vi "Lab Panel V5.11.vi"() -> ()   [LabVIEW 2013] (continued)
                  frame #0 {
                    n2509 = Merge Signals(w4745, w4744) -> (→"LAB01 AMPS":dynamicdata)
                    n2510 = Merge Signals(w4742, w4741) -> (→"LAB01 VOLTS":dynamicdata)
                    n2511 = Merge Signals(w4722, w4721) -> (→"LAB03 VOLTS":dynamicdata)
                    n2512 = Merge Signals(w4739, w4738, w4737, w4736) -> (→"LAB01 deg C":dynamicdata)
                    n2513 = Merge Signals(w4735, w4734) -> (→"LAB02 AMPS":dynamicdata)
                    n2514 = Merge Signals(w4728, w4727, w4726, w4725) -> (→"LAB02 deg C":dynamicdata)
                    n2515 = Merge Signals(w4720, w4719, w4718, w4717) -> (→"LAB03 deg C":dynamicdata)
                    n2516 = Merge Signals(w4732, w4731) -> (→"LAB02 VOLTS":dynamicdata)
                    n2517 = Merge Signals(w4724, w4723) -> (→"LAB03 AMPS":dynamicdata)
                  }
                  frame #1 {
                    n2518 = Merge Signals(w4755, w4754) -> (→"LAB05 VOLTS":dynamicdata)
                    n2519 = Merge Signals(w4768, w4767) -> (→"LAB04 AMPS":dynamicdata)
                    n2520 = Merge Signals(w4757, w4756) -> (→"LAB05 AMPS":dynamicdata)
                    n2521 = Merge Signals(w4753, w4752, w4751, w4750) -> (→"LAB05 deg C":dynamicdata)
                    n2522 = Merge Signals(w4764, w4763, w4762, w4761) -> (→"LAB04 deg C":dynamicdata)
                    n2523 = Merge Signals(w4766, w4765) -> (→"LAB04 VOLTS":dynamicdata)
                  }
                  frame #2 {
                    n2524 = local read "LAB05 VOLTS"() -> (w4776:dynamicdata)
                    n2525 = local read "LAB04 VOLTS"() -> (w4777:dynamicdata)
                    n2526 = local read "LAB02 VOLTS"() -> (w4779:dynamicdata)
                    n2527 = local read "LAB03 VOLTS"() -> (w4778:dynamicdata)
                    n2528 = local read "LAB05 AMPS"() -> (w4782:dynamicdata)
                    n2529 = local read "LAB01 VOLTS"() -> (w4780:dynamicdata)
                    n2530 = local read "LAB04 AMPS"() -> (w4783:dynamicdata)
                    n2531 = local read "LAB03 AMPS"() -> (w4784:dynamicdata)
                    n2532 = local read "LAB03 deg C"() -> (w4772:dynamicdata)
                    n2533 = local read "LAB02 AMPS"() -> (w4785:dynamicdata)
                    n2534 = local read "LAB04 deg C"() -> (w4771:dynamicdata)
                    n2535 = local read "LAB05 deg C"() -> (w4770:dynamicdata)
                    n2536 = local read "LAB02 deg C"() -> (w4773:dynamicdata)
                    n2537 = local read "LAB01 deg C"() -> (w4774:dynamicdata)
                    n2538 = local read "LAB01 AMPS"() -> (w4786:dynamicdata)
                    n2539 = Merge Signals(w4774, w4773, w4772, w4771, w4770) -> (w4769:dynamicdata)
                    n2540 = Merge Signals(w4786, w4785, w4784, w4783, w4782) -> (w4781:dynamicdata)
                    n2541 = Merge Signals(w4780, w4779, w4778, w4777, w4776) -> (w4775:dynamicdata)
                    n2542 = global write "Global display 3.vi" "graph volts"(w4775) -> ()
                    n2543 = global write "Global display 3.vi" "graph deg C"(w4769) -> ()
                    n2544 = global write "Global display 3.vi" "graph amps"(w4781) -> ()
                  }
                }
              }
            }
          }
          frame #14 {
            # "check for amps fail"
            # "check for cycle test & temperature rise fail conditions"
            n2545 = local read "on loops"() -> (w4813:dbl)
            n2546 = local read "jig cycle"() -> (w4810:dbl)
            n2547 = local read "jig cycle"() -> (w4815:dbl)
            n2548 = Add(x=w4813, y=3.0) -> (x+y=w4811:dbl)
            n2549 = Equal?(x=w4810, y=w4811) -> (x = y?=w4806:bool)
            n2550 = local read "Fail Loops"() -> (w4787:dbl)
            n2551 = Equal?(x=w4815, y=1.0) -> (x = y?=w4808:bool)
            n2552 = global write "Global 1.vi" "fail count"(w4787) -> ()
            n2553 = stacked-sequence {
              tunnel: w4809 -> [w4818 _ _ _ _ _ _ _ _ _]
              tunnel: w4808 -> [w4819 w4839 w4859 w4879 w4899 w4919 w4939 w4959 w4979 w4999]
              tunnel: w4807 -> [w4816 _ _ _ _ _ _ _ _ _]
              tunnel: w4806 -> [w4817 w4838 w4858 w4878 w4898 w4918 w4938 w4958 w4978 w4998]
              tunnel: w4805 -> [_ w4837 _ _ _ _ _ _ _ _]
              tunnel: w4804 -> [_ w4836 _ _ _ _ _ _ _ _]
              tunnel: w4803 -> [_ _ w4857 _ _ _ _ _ _ _]
              tunnel: w4802 -> [_ _ w4856 _ _ _ _ _ _ _]
              tunnel: w4801 -> [_ _ _ w4877 _ _ _ _ _ _]
              tunnel: w4800 -> [_ _ _ w4876 _ _ _ _ _ _]
              tunnel: w4799 -> [_ _ _ _ w4897 _ _ _ _ _]
              tunnel: w4798 -> [_ _ _ _ w4896 _ _ _ _ _]
              tunnel: w4797 -> [_ _ _ _ _ w4917 _ _ _ _]
              tunnel: w4796 -> [_ _ _ _ _ w4916 _ _ _ _]
              tunnel: w4795 -> [_ _ _ _ _ _ w4937 _ _ _]
              tunnel: w4794 -> [_ _ _ _ _ _ w4936 _ _ _]
              tunnel: w4793 -> [_ _ _ _ _ _ _ w4957 _ _]
              tunnel: w4792 -> [_ _ _ _ _ _ _ w4956 _ _]
              tunnel: w4791 -> [_ _ _ _ _ _ _ _ w4977 _]
              tunnel: w4790 -> [_ _ _ _ _ _ _ _ w4976 _]
              tunnel: w4789 -> [_ _ _ _ _ _ _ _ _ w4997]
              tunnel: w4788 -> [_ _ _ _ _ _ _ _ _ w4996]
              frame #0 {
                # "LAB01-1"
                n2554 = case shown="True" w4816 {
                  tunnel: w4819 -> [_ w4832]
                  tunnel: w4818 -> [_ w4829]
                  tunnel: w4817 -> [_ w4828]
                  frame False {
                  }
                  frame True {
                    n2555 = local read "TEMP START LAB01-1"() -> (w4834:cluster{"TL":dbl, "TN":dbl})
                    n2556 = local read "RESULT LAB01-1"() -> (w4823:bool)
                    n2557 = local read "FAIL LAB01-1"() -> (w4826:cluster{"LO":dbl, "HI":dbl})
                    n2558 = local read "TDMS LAB01-1"() -> (w4833:refnum<k34>)
                    n2559 = local read "SET LAB01-1"() -> (w4830:T5)
                    n2560 = local read "DISP LAB01-1"() -> (w4831:T4)
                    n2561 = local read "SIG LAB01-1"() -> (w4835:T2)
                    n2562 = Bundle("FAIL LAB01-1"=w4826, "SIG LAB01-1"=w4835, "TEMP START LAB01-1"=w4834, "DISP LAB01-1"=w4831, "SET LAB01-1"=w4830, "TDMS LAB01-1"=w4833) -> (w4820:T32)  [unwired: 1 in]
                    n2563 = call "sub vi - cycle&temp fail v7.vi"("Amps Lo?"=w4832, "Input Cluster"=w4820, "SELECT"=w4829, "Amps Hi?"=w4828, "Result In"=w4823) -> ("(FAIL) out"=w4825:cluster{"FAIL LO":dbl, "FAIL HI":dbl}, "(DISP) out"=w4821:T4, "T-RISE"=w4822:cluster{"T-RISE (L)":dbl, "T-RISE (N)":dbl}, "Result Out"=w4824:bool, "file error"=w4827:errorcluster)  [unwired: 10 in]
                    n2564 = local write "TEMP RISE LAB01-1"(w4822) -> ()
                    n2565 = local write "FAIL LAB01-1"(w4825) -> ()
                    n2566 = local write "DISP LAB01-1"(w4821) -> ()
                    n2567 = local write "RESULT LAB01-1"(w4824) -> ()
                    n2568 = local write "data file error"(w4827) -> ()
                  }
                }
              }
              frame #1 {
                # "LAB01-2"
                n2569 = case shown="True" w4837 {
                  tunnel: w4839 -> [_ w4852]
                  tunnel: w4836 -> [_ w4849]
                  tunnel: w4838 -> [_ w4848]
                  frame False {
                  }
                  frame True {
                    n2570 = local read "TEMP START LAB01-2"() -> (w4854:cluster{"TL":dbl, "TN":dbl})
                    n2571 = local read "FAIL LAB01-2"() -> (w4845:cluster{"LO":dbl, "HI":dbl})
                    n2572 = local read "TDMS LAB01-2"() -> (w4853:refnum<k34>)
                    n2573 = local read "SET LAB01-2"() -> (w4850:T5)
                    n2574 = local read "DISP LAB01-2"() -> (w4851:T4)
                    n2575 = local read "RESULT LAB01-2"() -> (w4842:bool)
                    n2576 = local read "SIG LAB01-2"() -> (w4855:T2)
                    n2577 = Bundle("FAIL LAB01-2"=w4845, "SIG LAB01-2"=w4855, "TEMP START LAB01-2"=w4854, "DISP LAB01-2"=w4851, "SET LAB01-2"=w4850, "TDMS LAB01-2"=w4853) -> (w4840:T33)  [unwired: 1 in]
                    n2578 = call "sub vi - cycle&temp fail v7.vi"("Amps Lo?"=w4852, "Input Cluster"=w4840, "SELECT"=w4849, "Amps Hi?"=w4848, "Result In"=w4842) -> ("(FAIL) out"=w4844:cluster{"FAIL LO":dbl, "FAIL HI":dbl}, "(DISP) out"=w4847:T4, "T-RISE"=w4841:cluster{"T-RISE (L)":dbl, "T-RISE (N)":dbl}, "Result Out"=w4843:bool, "file error"=w4846:errorcluster)  [unwired: 10 in]
                    n2579 = local write "TEMP RISE LAB01-2"(w4841) -> ()
                    n2580 = local write "FAIL LAB01-2"(w4844) -> ()
                    n2581 = local write "DISP LAB01-2"(w4847) -> ()
                    n2582 = local write "RESULT LAB01-2"(w4843) -> ()
                    n2583 = local write "data file error"(w4846) -> ()
                  }
                }
              }
              frame #2 {
                # "LAB02-1"
                n2584 = case shown="True" w4857 {
                  tunnel: w4859 -> [_ w4872]
                  tunnel: w4856 -> [_ w4869]
                  tunnel: w4858 -> [_ w4868]
                  frame False {
                  }
                  frame True {
                    n2585 = local read "TEMP START LAB02-1"() -> (w4874:cluster{"TL":dbl, "TN":dbl})
                    n2586 = local read "FAIL LAB02-1"() -> (w4865:cluster{"LO":dbl, "HI":dbl})
                    n2587 = local read "TDMS LAB02-1"() -> (w4873:refnum<k34>)
                    n2588 = local read "SET LAB02-1"() -> (w4870:T5)
                    n2589 = local read "DISP LAB02-1"() -> (w4871:T4)
                    n2590 = local read "SIG LAB02-1"() -> (w4875:T2)
                    n2591 = local read "RESULT LAB02-1"() -> (w4862:bool)
                    n2592 = Bundle("FAIL LAB02-1"=w4865, "SIG LAB02-1"=w4875, "TEMP START LAB02-1"=w4874, "DISP LAB02-1"=w4871, "SET LAB02-1"=w4870, "TDMS LAB02-1"=w4873) -> (w4860:T34)  [unwired: 1 in]
                    n2593 = call "sub vi - cycle&temp fail v7.vi"("Amps Lo?"=w4872, "Input Cluster"=w4860, "SELECT"=w4869, "Amps Hi?"=w4868, "Result In"=w4862) -> ("(FAIL) out"=w4864:cluster{"FAIL LO":dbl, "FAIL HI":dbl}, "(DISP) out"=w4867:T4, "T-RISE"=w4861:cluster{"T-RISE (L)":dbl, "T-RISE (N)":dbl}, "Result Out"=w4863:bool, "file error"=w4866:errorcluster)  [unwired: 10 in]
                    n2594 = local write "TEMP RISE LAB02-1"(w4861) -> ()
                    n2595 = local write "FAIL LAB02-1"(w4864) -> ()
                    n2596 = local write "DISP LAB02-1"(w4867) -> ()
                    n2597 = local write "RESULT LAB02-1"(w4863) -> ()
                    n2598 = local write "data file error"(w4866) -> ()
                  }
                }
              }
              frame #3 {
                # "LAB02-2"
                n2599 = case shown="True" w4877 {
                  tunnel: w4879 -> [_ w4892]
                  tunnel: w4876 -> [_ w4889]
                  tunnel: w4878 -> [_ w4888]
                  frame False {
                  }
                  frame True {
                    n2600 = local read "TEMP START LAB02-2"() -> (w4894:cluster{"TL":dbl, "TN":dbl})
                    n2601 = local read "FAIL LAB02-2"() -> (w4885:cluster{"LO":dbl, "HI":dbl})
                    n2602 = local read "TDMS LAB02-2"() -> (w4893:refnum<k34>)
                    n2603 = local read "SET LAB02-2"() -> (w4890:T5)
                    n2604 = local read "DISP LAB02-2"() -> (w4891:T4)
                    n2605 = local read "SIG LAB02-2"() -> (w4895:T2)
                    n2606 = local read "RESULT LAB02-2"() -> (w4882:bool)
                    n2607 = Bundle("FAIL LAB02-2"=w4885, "SIG LAB02-2"=w4895, "TEMP START LAB02-2"=w4894, "DISP LAB02-2"=w4891, "SET LAB02-2"=w4890, "TDMS LAB02-2"=w4893) -> (w4880:T35)  [unwired: 1 in]
                    n2608 = call "sub vi - cycle&temp fail v7.vi"("Amps Lo?"=w4892, "Input Cluster"=w4880, "SELECT"=w4889, "Amps Hi?"=w4888, "Result In"=w4882) -> ("(FAIL) out"=w4884:cluster{"FAIL LO":dbl, "FAIL HI":dbl}, "(DISP) out"=w4887:T4, "T-RISE"=w4881:cluster{"T-RISE (L)":dbl, "T-RISE (N)":dbl}, "Result Out"=w4883:bool, "file error"=w4886:errorcluster)  [unwired: 10 in]
                    n2609 = local write "TEMP RISE LAB02-2"(w4881) -> ()
                    n2610 = local write "FAIL LAB02-2"(w4884) -> ()
                    n2611 = local write "DISP LAB02-2"(w4887) -> ()
                    n2612 = local write "RESULT LAB02-2"(w4883) -> ()
                    n2613 = local write "data file error"(w4886) -> ()
                  }
                }
              }
              frame #4 {
                # "LAB03-1"
                n2614 = case shown="True" w4897 {
                  tunnel: w4899 -> [_ w4912]
                  tunnel: w4896 -> [_ w4909]
                  tunnel: w4898 -> [_ w4908]
                  frame False {
                  }
                  frame True {
                    n2615 = local read "TEMP START LAB03-1"() -> (w4914:cluster{"TL":dbl, "TN":dbl})
                    n2616 = local read "FAIL LAB03-1"() -> (w4905:cluster{"LO":dbl, "HI":dbl})
                    n2617 = local read "TDMS LAB03-1"() -> (w4913:refnum<k34>)
                    n2618 = local read "SET LAB03-1"() -> (w4910:T5)
                    n2619 = local read "DISP LAB03-1"() -> (w4911:T4)
                    n2620 = local read "SIG LAB03-1"() -> (w4915:T2)
                    n2621 = local read "RESULT LAB03-1"() -> (w4902:bool)
                    n2622 = Bundle("FAIL LAB03-1"=w4905, "SIG LAB03-1"=w4915, "TEMP START LAB03-1"=w4914, "DISP LAB03-1"=w4911, "SET LAB03-1"=w4910, "TDMS LAB03-1"=w4913) -> (w4900:T36)  [unwired: 1 in]
                    n2623 = call "sub vi - cycle&temp fail v7.vi"("Amps Lo?"=w4912, "Input Cluster"=w4900, "SELECT"=w4909, "Amps Hi?"=w4908, "Result In"=w4902) -> ("(FAIL) out"=w4904:cluster{"FAIL LO":dbl, "FAIL HI":dbl}, "(DISP) out"=w4907:T4, "T-RISE"=w4901:cluster{"T-RISE (L)":dbl, "T-RISE (N)":dbl}, "Result Out"=w4903:bool, "file error"=w4906:errorcluster)  [unwired: 10 in]
                    n2624 = local write "TEMP RISE LAB03-1"(w4901) -> ()
                    n2625 = local write "FAIL LAB03-1"(w4904) -> ()
                    n2626 = local write "DISP LAB03-1"(w4907) -> ()
                    n2627 = local write "RESULT LAB03-1"(w4903) -> ()
                    n2628 = local write "data file error"(w4906) -> ()
                  }
                }
              }
              frame #5 {
                # "LAB03-2"
                n2629 = case shown="True" w4917 {
                  tunnel: w4919 -> [_ w4932]
                  tunnel: w4916 -> [_ w4929]
                  tunnel: w4918 -> [_ w4928]
                  frame False {
                  }
                  frame True {
                    n2630 = local read "TEMP START LAB03-2"() -> (w4934:cluster{"TL":dbl, "TN":dbl})
                    n2631 = local read "FAIL LAB03-2"() -> (w4925:cluster{"LO":dbl, "HI":dbl})
                    n2632 = local read "TDMS LAB03-2"() -> (w4933:refnum<k34>)
                    n2633 = local read "SET LAB03-2"() -> (w4930:T5)
                    n2634 = local read "DISP LAB03-2"() -> (w4931:T4)
                    n2635 = local read "RESULT LAB03-2"() -> (w4922:bool)
                    n2636 = local read "SIG LAB03-2"() -> (w4935:T2)
                    n2637 = Bundle("FAIL LAB03-2"=w4925, "SIG LAB03-2"=w4935, "TEMP START LAB03-2"=w4934, "DISP LAB03-2"=w4931, "SET LAB03-2"=w4930, "TDMS LAB03-2"=w4933) -> (w4920:T37)  [unwired: 1 in]
                    n2638 = call "sub vi - cycle&temp fail v7.vi"("Amps Lo?"=w4932, "Input Cluster"=w4920, "SELECT"=w4929, "Amps Hi?"=w4928, "Result In"=w4922) -> ("(FAIL) out"=w4924:cluster{"FAIL LO":dbl, "FAIL HI":dbl}, "(DISP) out"=w4927:T4, "T-RISE"=w4921:cluster{"T-RISE (L)":dbl, "T-RISE (N)":dbl}, "Result Out"=w4923:bool, "file error"=w4926:errorcluster)  [unwired: 10 in]
                    n2639 = local write "FAIL LAB03-2"(w4924) -> ()
                    n2640 = local write "TEMP RISE LAB03-2"(w4921) -> ()
                    n2641 = local write "DISP LAB03-2"(w4927) -> ()
                    n2642 = local write "RESULT LAB03-2"(w4923) -> ()
                    n2643 = local write "data file error"(w4926) -> ()
                  }
                }
              }
              frame #6 {
                # "LAB04-1"
                n2644 = case shown="True" w4937 {
                  tunnel: w4939 -> [_ w4952]
                  tunnel: w4936 -> [_ w4949]
                  tunnel: w4938 -> [_ w4948]
                  frame False {
                  }
                  frame True {
                    n2645 = local read "TEMP START LAB04-1"() -> (w4954:cluster{"TL":dbl, "TN":dbl})
                    n2646 = local read "FAIL LAB04-1"() -> (w4945:cluster{"LO":dbl, "HI":dbl})
                    n2647 = local read "TDMS LAB04-1"() -> (w4953:refnum<k34>)
                    n2648 = local read "SET LAB04-1"() -> (w4950:T5)
                    n2649 = local read "DISP LAB04-1"() -> (w4951:T4)
                    n2650 = local read "SIG LAB04-1"() -> (w4955:T2)
                    n2651 = local read "RESULT LAB04-1"() -> (w4942:bool)
                    n2652 = Bundle("FAIL LAB04-1"=w4945, "SIG LAB04-1"=w4955, "TEMP START LAB04-1"=w4954, "DISP LAB04-1"=w4951, "SET LAB04-1"=w4950, "TDMS LAB04-1"=w4953) -> (w4940:T38)  [unwired: 1 in]
                    n2653 = call "sub vi - cycle&temp fail v7.vi"("Amps Lo?"=w4952, "Input Cluster"=w4940, "SELECT"=w4949, "Amps Hi?"=w4948, "Result In"=w4942) -> ("(FAIL) out"=w4944:cluster{"FAIL LO":dbl, "FAIL HI":dbl}, "(DISP) out"=w4947:T4, "T-RISE"=w4941:cluster{"T-RISE (L)":dbl, "T-RISE (N)":dbl}, "Result Out"=w4943:bool, "file error"=w4946:errorcluster)  [unwired: 10 in]
                    n2654 = local write "TEMP RISE LAB04-1"(w4941) -> ()
                    n2655 = local write "FAIL LAB04-1"(w4944) -> ()
                    n2656 = local write "DISP LAB04-1"(w4947) -> ()
                    n2657 = local write "RESULT LAB04-1"(w4943) -> ()
                    n2658 = local write "data file error"(w4946) -> ()
                  }
                }
              }
              frame #7 {
                # "LAB04-2"
                n2659 = case shown="True" w4957 {
                  tunnel: w4959 -> [_ w4972]
                  tunnel: w4956 -> [_ w4969]
                  tunnel: w4958 -> [_ w4968]
                  frame False {
                  }
                  frame True {
                    n2660 = local read "TEMP START LAB04-2"() -> (w4974:cluster{"TL":dbl, "TN":dbl})
                    n2661 = local read "FAIL LAB04-2"() -> (w4965:cluster{"LO":dbl, "HI":dbl})
                    n2662 = local read "TDMS LAB04-2"() -> (w4973:refnum<k34>)
                    n2663 = local read "SET LAB04-2"() -> (w4970:T5)
                    n2664 = local read "DISP LAB04-2"() -> (w4971:T4)
                    n2665 = local read "SIG LAB04-2"() -> (w4975:T2)
                    n2666 = local read "RESULT LAB04-2"() -> (w4962:bool)
                    n2667 = Bundle("FAIL LAB04-2"=w4965, "SIG LAB04-2"=w4975, "TEMP START LAB04-2"=w4974, "DISP LAB04-2"=w4971, "SET LAB04-2"=w4970, "TDMS LAB04-2"=w4973) -> (w4960:T39)  [unwired: 1 in]
                    n2668 = call "sub vi - cycle&temp fail v7.vi"("Amps Lo?"=w4972, "Input Cluster"=w4960, "SELECT"=w4969, "Amps Hi?"=w4968, "Result In"=w4962) -> ("(FAIL) out"=w4964:cluster{"FAIL LO":dbl, "FAIL HI":dbl}, "(DISP) out"=w4967:T4, "T-RISE"=w4961:cluster{"T-RISE (L)":dbl, "T-RISE (N)":dbl}, "Result Out"=w4963:bool, "file error"=w4966:errorcluster)  [unwired: 10 in]
                    n2669 = local write "TEMP RISE LAB04-2"(w4961) -> ()
                    n2670 = local write "FAIL LAB04-2"(w4964) -> ()
                    n2671 = local write "DISP LAB04-2"(w4967) -> ()
                    n2672 = local write "RESULT LAB04-2"(w4963) -> ()
                    n2673 = local write "data file error"(w4966) -> ()
                  }
                }
              }
              frame #8 {
                # "LAB05-1"
                n2674 = case shown="True" w4977 {
                  tunnel: w4979 -> [_ w4992]
                  tunnel: w4976 -> [_ w4989]
                  tunnel: w4978 -> [_ w4988]
                  frame False {
                  }
                  frame True {
                    n2675 = local read "TEMP START LAB05-1"() -> (w4994:cluster{"TL":dbl, "TN":dbl})
                    n2676 = local read "FAIL LAB05-1"() -> (w4985:cluster{"LO":dbl, "HI":dbl})
                    n2677 = local read "TDMS LAB05-1"() -> (w4993:refnum<k34>)
                    n2678 = local read "SET LAB05-1"() -> (w4990:T5)
                    n2679 = local read "DISP LAB05-1"() -> (w4991:T4)
                    n2680 = local read "SIG LAB05-1"() -> (w4995:T2)
                    n2681 = local read "RESULT LAB05-1"() -> (w4982:bool)
                    n2682 = Bundle("FAIL LAB05-1"=w4985, "SIG LAB05-1"=w4995, "TEMP START LAB05-1"=w4994, "DISP LAB05-1"=w4991, "SET LAB05-1"=w4990, "TDMS LAB05-1"=w4993) -> (w4980:T40)  [unwired: 1 in]
                    n2683 = call "sub vi - cycle&temp fail v7.vi"("Amps Lo?"=w4992, "Input Cluster"=w4980, "SELECT"=w4989, "Amps Hi?"=w4988, "Result In"=w4982) -> ("(FAIL) out"=w4984:cluster{"FAIL LO":dbl, "FAIL HI":dbl}, "(DISP) out"=w4987:T4, "T-RISE"=w4981:cluster{"T-RISE (L)":dbl, "T-RISE (N)":dbl}, "Result Out"=w4983:bool, "file error"=w4986:errorcluster)  [unwired: 10 in]
                    n2684 = local write "TEMP RISE LAB05-1"(w4981) -> ()
                    n2685 = local write "FAIL LAB05-1"(w4984) -> ()
                    n2686 = local write "DISP LAB05-1"(w4987) -> ()
                    n2687 = local write "RESULT LAB05-1"(w4983) -> ()
                    n2688 = local write "data file error"(w4986) -> ()
                  }
                }
              }
              frame #9 {
                # "LAB05-2"
                n2689 = case shown="True" w4997 {
                  tunnel: w4999 -> [_ w5012]
                  tunnel: w4996 -> [_ w5009]
                  tunnel: w4998 -> [_ w5008]
                  frame False {
                  }
                  frame True {
                    n2690 = local read "TEMP START LAB05-2"() -> (w5014:cluster{"TL":dbl, "TN":dbl})
                    n2691 = local read "FAIL LAB05-2"() -> (w5005:cluster{"LO":dbl, "HI":dbl})
                    n2692 = local read "TDMS LAB05-2"() -> (w5013:refnum<k34>)
                    n2693 = local read "SET LAB05-2"() -> (w5010:T5)
                    n2694 = local read "DISP LAB05-2"() -> (w5011:T4)
                    n2695 = local read "SIG LAB05-2"() -> (w5015:T2)
                    n2696 = local read "RESULT LAB05-2"() -> (w5002:bool)
                    n2697 = Bundle("FAIL LAB05-2"=w5005, "SIG LAB05-2"=w5015, "TEMP START LAB05-2"=w5014, "DISP LAB05-2"=w5011, "SET LAB05-2"=w5010, "TDMS LAB05-2"=w5013) -> (w5000:T41)  [unwired: 1 in]
                    n2698 = call "sub vi - cycle&temp fail v7.vi"("Amps Lo?"=w5012, "Input Cluster"=w5000, "SELECT"=w5009, "Amps Hi?"=w5008, "Result In"=w5002) -> ("(FAIL) out"=w5004:cluster{"FAIL LO":dbl, "FAIL HI":dbl}, "(DISP) out"=w5007:T4, "T-RISE"=w5001:cluster{"T-RISE (L)":dbl, "T-RISE (N)":dbl}, "Result Out"=w5003:bool, "file error"=w5006:errorcluster)  [unwired: 10 in]
                    n2699 = local write "TEMP RISE LAB05-2"(w5001) -> ()
                    n2700 = local write "FAIL LAB05-2"(w5004) -> ()
                    n2701 = local write "DISP LAB05-2"(w5007) -> ()
                    n2702 = local write "RESULT LAB05-2"(w5003) -> ()
                    n2703 = local write "data file error"(w5006) -> ()
                  }
                }
              }
            }
          }
          frame #15 {
            # "run calibration routine"
            n2704 = local read "SET (cal)"() -> (w5016:bool)
            n2705 = case shown="True" w5016 {
              frame False {
              }
              frame True {
                n2706 = stacked-sequence {
                  seq-local: [w5017 _ _] -> [_ w5019 _]
                  frame #0 {
                    n2707 = call "CALIBRATION PASSWORD"() -> ("PASSWORD"=w5017:string)  [unwired: 17 in, 2 out]
                  }
                  frame #1 {
                    n2708 = Equal?(x=w5019, y="7777") -> (x = y?=w5018:bool)
                    n2709 = case shown="True" w5018 {
                      frame False {
                      }
                      frame True {
                        n2710 = stacked-sequence {
                          frame #0 {
                            n2711 = local read "Temp Test Cal"() -> (w5021:dbl)
                            n2712 = call "sub vi - calibration v1.vi"("Temp Test Cal"=w5021) -> ()  [unwired: 11 in]
                          }
                          frame #1 {
                            n2713 = call "sub vi - get calibration values v1.vi"() -> ("TEMP REF CAL"=w5022:dbl, "LAB01 (CAL)"=w5027:T14, "LAB02 (CAL)"=w5026:T15, "LAB03 (CAL)"=w5025:T14, "LAB04 (CAL)"=w5024:T14, "calibration file error out"=w5028:errorcluster, "LAB05 (CAL)"=w5023:T14)  [unwired: 9 in]
                            n2714 = local write "TEMP REF cal"(w5022) -> ()
                            n2715 = local write "cal file error out"(w5028) -> ()
                            n2716 = local write "CAL LAB04"(w5024) -> ()
                            n2717 = local write "CAL LAB05"(w5023) -> ()
                            n2718 = local write "CAL LAB01"(w5027) -> ()
                            n2719 = local write "CAL LAB02"(w5026) -> ()
                            n2720 = local write "CAL LAB03"(w5025) -> ()
                          }
                        }
                      }
                    }
                  }
                  frame #2 {
                    n2721 = local write "SET (cal)"(FALSE) -> ()
                  }
                }
              }
            }
          }
          frame #16 {
            # "save certain settings to file"
            n2722 = String To Path(string="c:\\crabtree\\Set Up\\") -> (path=w5031:path)
            n2723 = Build Path(base path=w5031, name or relative path="settings.bin") -> (appended path=w5033:path)
            n2724 = Build Path(base path=w5031, name or relative path="mail.bin") -> (appended path=w5030:path)
            n2725 = Create Folder(path (use dialog)=w5031) -> (error out=w5036:errorcluster)  [unwired: 2 in, 2 out]
            n2726 = call <vilib>:"Clear Errors.vi"("error in (no error)"=w5036) -> ()  [unwired: 6 in, 1 out]
            n2727 = stacked-sequence {
              seq-local: [w5048 _] -> [_ w5061]
              tunnel: w5033 -> [_ w5062]
              tunnel: w5030 -> [_ w5060]
              frame #0 {
                n2728 = local read "C drive data root dir"() -> (w5047:path)
                n2729 = local read "Select COM port"() -> (w5044:refnum<visa-resource-name>)
                n2730 = local read "Network Directory"() -> (w5053:path)
                n2731 = local read "SET LAB05-2"() -> (w5052:T5)
                n2732 = local read "SET LAB05-1"() -> (w5051:T5)
                n2733 = local read "SET LAB04-2"() -> (w5050:T5)
                n2734 = local read "SET LAB03-2"() -> (w5054:T5)
                n2735 = local read "SET LAB04-1"() -> (w5049:T5)
                n2736 = local read "SET LAB03-1"() -> (w5055:T5)
                n2737 = local read "SET LAB02-2"() -> (w5056:T5)
                n2738 = local read "SET LAB02-1"() -> (w5057:T5)
                n2739 = local read "Temp Delay Lps"() -> (w5043:dbl)
                n2740 = local read "Amps Fail level"() -> (w5039:dbl)
                n2741 = local read "SET LAB01-2"() -> (w5058:T5)
                n2742 = local read "Temp Test Cal"() -> (w5040:dbl)
                n2743 = local read "SET LAB01-1"() -> (w5059:T5)
                n2744 = local read "Mail Test File To:"() -> (w5038:string)
                n2745 = local read "Temp Value"() -> (w5042:dbl)
                n2746 = local read "Fail Loops"() -> (w5041:dbl)
                n2747 = local read "Mail Test Fail"() -> (w5037:bool)
                n2748 = local read "RATE (Hz)"() -> (w5046:dbl)
                n2749 = local read "SAMPLES"() -> (w5045:dbl)
                n2750 = Bundle("SET LAB01-1"=w5059, "SET LAB01-2"=w5058, "SET LAB02-1"=w5057, "SET LAB02-2"=w5056, "SET LAB03-1"=w5055, "SET LAB03-2"=w5054, "SET LAB04-1"=w5049, "SET LAB04-2"=w5050, "SET LAB05-1"=w5051, "SET LAB05-2"=w5052, "Network Directory"=w5053, "C drive data root dir"=w5047, "RATE (Hz)"=w5046, "SAMPLES"=w5045, "Select COM port"=w5044, "Temp Delay Lps"=w5043, "Temp Value"=w5042, "Fail Loops"=w5041, "Temp Test Cal"=w5040, "Amps Fail level"=w5039, "Mail Test File To:"=w5038, "Mail Test Fail"=w5037) -> (w5048:T22)  [unwired: 1 in]
              }
              frame #1 {
                n2751 = event shown="[1] \"SET LAB01-1\", \"SET LAB01-2\", \"SET LAB02-1\", \"SET LAB02-2\", \"SET LAB03-1\", \"SET LAB03-2\", \"SET LAB04-1\", \"SET LAB04-2\", \"SET LAB05-1\", \"SET LAB05-2\", \"Network Directory\", \"C drive data root dir\", \"RATE (Hz)\", \"SAMPLES\", \"Select COM port\", \"Temp Delay Lps\", \"Temp Value\", \"Fail Loops\", \"Temp Test Cal\", \"Amps Fail level\", \"Mail Test File To:\", \"Mail Test Fail\": Value Change" {
                  selector: _ -> [_ _ _]
                  dyn-events: _ -> [_ _ _]
                  timeout: 10.0 -> [_ _ _]
                  tunnel: w5062 -> [_ w5064 _]
                  tunnel: w5061 -> [_ w5065 _]
                  tunnel: w5060 -> [_ _ w5076]
                  event Timeout {
                    n2752 = event-data() -> ()  [unwired: 1 in, 3 out]
                  }
                  event "SET LAB01-1", "SET LAB01-2", "SET LAB02-1", "SET LAB02-2", "SET LAB03-1", "SET LAB03-2", "SET LAB04-1", "SET LAB04-2", "SET LAB05-1", "SET LAB05-2", "Network Directory", "C drive data root dir", "RATE (Hz)", "SAMPLES", "Select COM port", "Temp Delay Lps", "Temp Value", "Fail Loops", "Temp Test Cal", "Amps Fail level", "Mail Test File To:", "Mail Test Fail": Value Change {
                    n2753 = event-data() -> ()  [unwired: 1 in, 6 out]
                    n2754 = Open/Create/Replace File(file path (use dialog)=w5064, operation (0:open)=T21."replace or create") -> (refnum out=w5070:refnum<file>, error out=w5069:errorcluster)  [unwired: 4 in, 1 out]
                    n2755 = Write to Binary File(file (use dialog)=w5070, data=w5065, error in=w5069) -> (refnum out=w5068:refnum<file>, error out=w5067:errorcluster)  [unwired: 3 in, 1 out]
                    n2756 = Close File(refnum=w5068, error in=w5067) -> (error out=w5066:errorcluster)  [unwired: 1 out]
                    n2757 = local write "data file error"(w5066) -> ()
                  }
                  event "MAIL SETTINGS.OUT SERVER ADDRESS", "MAIL SETTINGS.FROM ACCOUNT", "MAIL SETTINGS.USER NAME", "MAIL SETTINGS.PASSWORD", "Auto Mail Send", "TO (string):": Value Change {
                    n2758 = event-data() -> ()  [unwired: 1 in, 6 out]
                    n2759 = local read "MAIL SETTINGS"() -> (w5075:T7)
                    n2760 = local read "Auto Mail Send"() -> (w5073:bool)
                    n2761 = local read "TO (string):"() -> (w5072:string)
                    n2762 = Open/Create/Replace File(file path (use dialog)=w5076, operation (0:open)=T21."replace or create") -> (refnum out=w5081:refnum<file>, error out=w5080:errorcluster)  [unwired: 4 in, 1 out]
                    n2763 = Bundle("MAIL SETTINGS"=w5075, "Auto Mail Send"=w5073, "TO (string):"=w5072) -> (w5074:T42)  [unwired: 1 in]
                    n2764 = Write to Binary File(file (use dialog)=w5081, data=w5074, error in=w5080) -> (refnum out=w5079:refnum<file>, error out=w5078:errorcluster)  [unwired: 3 in, 1 out]
                    n2765 = Close File(refnum=w5079, error in=w5078) -> (error out=w5077:errorcluster)  [unwired: 1 out]
                    n2766 = local write "data file error"(w5077) -> ()
                  }
                }
              }
            }
          }
          frame #17 {
            # "mail control"
            n2767 = local read "MAIL SETTINGS"() -> (w5098:T7)
            n2768 = local read "Auto Mail Send"() -> (w5084:bool)
            n2769 = Unbundle(w5098) -> ("OUT SERVER ADDRESS"=w5097:string, "FROM ACCOUNT"=w5096:string, "TEST MAIL"=w5095:bool)  [unwired: 4 out]
            n2770 = stacked-sequence {
              tunnel: "TO (string):" -> [_ w5137]
              tunnel: w5098 -> [w5103 w5136]
              tunnel: w5097 -> [w5102 w5135]
              tunnel: w5096 -> [w5101 w5134]
              tunnel: w5095 -> [w5100 _]
              tunnel: w5084 -> [_ w5133]
              tunnel: w5094 -> [_ w5132]
              tunnel: w5093 -> [_ w5131]
              tunnel: w5092 -> [_ w5130]
              tunnel: w5091 -> [_ w5129]
              tunnel: w5090 -> [_ w5128]
              tunnel: w5089 -> [_ w5127]
              tunnel: w5088 -> [_ w5126]
              tunnel: w5087 -> [_ w5125]
              tunnel: w5086 -> [_ w5124]
              tunnel: w5085 -> [_ w5123]
              tunnel: "TO (string):" -> [w5099 _]
              frame #0 {
                # "mail test"
                n2771 = case shown="True" w5100 {
                  tunnel: w5103 -> [_ w5107]
                  tunnel: w5099 -> [_ w5106]
                  tunnel: w5102 -> [_ w5105]
                  tunnel: w5101 -> [_ w5104]
                  frame False {
                  }
                  frame True {
                    n2772 = stacked-sequence {
                      seq-local: [_ _ w5117 _] -> [_ _ _ w5118]
                      tunnel: w5107 -> [w5110 _ _ w5122]
                      tunnel: w5106 -> [_ _ w5115 _]
                      tunnel: w5105 -> [_ _ w5113 _]
                      tunnel: w5104 -> [_ _ w5114 _]
                      frame #0 {
                        n2773 = Bundle(cluster=w5110, "TEST MAIL STATUS"="TEST START") -> (w5108:T7)  [unwired: 6 in]
                        n2774 = local write "MAIL SETTINGS"(w5108) -> ()
                      }
                      frame #1 {
                        n2775 = Wait (ms)(milliseconds to wait=500) -> ()  [unwired: 1 out]
                      }
                      frame #2 {
                        n2776 = call "sub vi - send mail v5.vi"("TO:"=w5115, "subject"="MAIL TEST FROM LAB PANEL", "from"=w5114, "out going server"=w5113, "message"="TEST MESSAGE") -> ("error out"=w5117:errorcluster)  [unwired: 10 in]
                      }
                      frame #3 {
                        n2777 = Bundle(cluster=w5122, "TEST MAIL"=FALSE, "TEST MAIL STATUS"="TEST END", "mail error"=w5118) -> (w5120:T7)  [unwired: 4 in]
                        n2778 = local write "MAIL SETTINGS"(w5120) -> ()
                      }
                    }
                  }
                }
              }
              frame #1 {
                # "mail report"
                n2779 = stacked-sequence {
                  seq-local: [_ w5180 _ _] -> [_ _ _ w5370]
                  seq-local: [_ _ w5283 _] -> [_ _ _ w5360]
                  seq-local: [w5147 _ _ _] -> [_ w5197 _ _]
                  seq-local: [w5146 _ _ _] -> [_ w5196 _ _]
                  seq-local: [w5144 _ _ _] -> [_ w5194 _ _]
                  seq-local: [w5145 _ _ _] -> [_ w5195 _ _]
                  seq-local: [w5143 _ _ _] -> [_ w5193 _ _]
                  seq-local: [w5142 _ _ _] -> [_ w5188 _ _]
                  seq-local: [w5141 _ _ _] -> [_ w5189 _ _]
                  seq-local: [w5140 _ _ _] -> [_ w5190 _ _]
                  seq-local: [w5139 _ _ _] -> [_ w5191 _ _]
                  seq-local: [w5138 _ _ _] -> [_ w5192 _ _]
                  tunnel: w5137 -> [_ _ _ w5371]
                  tunnel: w5136 -> [_ _ _ w5354]
                  tunnel: w5135 -> [_ _ _ w5368]
                  tunnel: w5134 -> [_ _ _ w5367]
                  tunnel: w5133 -> [w5178 _ _ w5362]
                  tunnel: w5132 -> [_ _ w5313 _]
                  tunnel: w5131 -> [_ _ w5310 _]
                  tunnel: w5130 -> [_ _ w5309 _]
                  tunnel: w5129 -> [_ _ w5308 _]
                  tunnel: w5128 -> [_ _ w5307 _]
                  tunnel: w5127 -> [_ _ w5306 _]
                  tunnel: w5126 -> [_ _ w5305 _]
                  tunnel: w5125 -> [_ _ w5304 _]
                  tunnel: w5124 -> [_ _ w5303 _]
                  tunnel: w5123 -> [_ _ w5302 _]
                  frame #0 {
                    n2780 = case shown="False" w5178 {
                      frame False {
                        n2781 = local write "mail control"("") -> ()
                      }
                      frame True {
                      }
                    }
                    n2782 = local read "SET LAB01-1"() -> (w5177:T5)
                    n2783 = local read "SET LAB01-2"() -> (w5176:T5)
                    n2784 = local read "SET LAB02-1"() -> (w5175:T5)
                    n2785 = local read "SET LAB02-2"() -> (w5174:T5)
                    n2786 = local read "SET LAB03-1"() -> (w5173:T5)
                    n2787 = local read "SET LAB04-1"() -> (w5171:T5)
                    n2788 = local read "SET LAB05-1"() -> (w5169:T5)
                    n2789 = local read "SET LAB03-2"() -> (w5172:T5)
                    n2790 = local read "SET LAB04-2"() -> (w5170:T5)
                    n2791 = local read "SET LAB05-2"() -> (w5168:T5)
                    n2792 = Unbundle(w5173) -> ("DESCRIPTION"=w5153:string)  [unwired: 4 out]
                    n2793 = Unbundle(w5172) -> ("DESCRIPTION"=w5152:string)  [unwired: 4 out]
                    n2794 = Unbundle(w5171) -> ("DESCRIPTION"=w5151:string)  [unwired: 4 out]
                    n2795 = Unbundle(w5168) -> ("DESCRIPTION"=w5148:string)  [unwired: 4 out]
                    n2796 = Unbundle(w5174) -> ("DESCRIPTION"=w5154:string)  [unwired: 4 out]
                    n2797 = Unbundle(w5170) -> ("DESCRIPTION"=w5150:string)  [unwired: 4 out]
                    n2798 = Unbundle(w5177) -> ("DESCRIPTION"=w5166:string)  [unwired: 4 out]
                    n2799 = Unbundle(w5175) -> ("DESCRIPTION"=w5155:string)  [unwired: 4 out]
                    n2800 = Unbundle(w5169) -> ("DESCRIPTION"=w5149:string)  [unwired: 4 out]
                    n2801 = Unbundle(w5176) -> ("DESCRIPTION"=w5156:string)  [unwired: 4 out]
                    n2802 = Concatenate Strings("[LAB05-2/", w5148) -> (w5138:string)
                    n2803 = Concatenate Strings("[LAB05-1/", w5149) -> (w5139:string)
                    n2804 = Concatenate Strings("[LAB04-2/", w5150) -> (w5140:string)
                    n2805 = Concatenate Strings("[LAB03-2/", w5152) -> (w5142:string)
                    n2806 = Concatenate Strings("[LAB04-1/", w5151) -> (w5141:string)
                    n2807 = Concatenate Strings("[LAB03-1/", w5153) -> (w5143:string)
                    n2808 = Concatenate Strings("[LAB01-2/", w5156) -> (w5146:string)
                    n2809 = Concatenate Strings("[LAB02-2/", w5154) -> (w5144:string)
                    n2810 = Concatenate Strings("[LAB01-1/", w5166) -> (w5147:string)
                    n2811 = Concatenate Strings("[LAB02-1/", w5155) -> (w5145:string)
                  }
                  frame #1 {
                    w5201 = "/"
                    w5202 = 2.0
                    n2812 = local read "DISP LAB01-2"() -> (w5281:T4)
                    n2813 = local read "DISP LAB01-1"() -> (w5282:T4)
                    n2814 = local read "DISP LAB02-1"() -> (w5280:T4)
                    n2815 = local read "DISP LAB03-2"() -> (w5277:T4)
                    n2816 = local read "DISP LAB02-2"() -> (w5279:T4)
                    n2817 = local read "DISP LAB03-1"() -> (w5278:T4)
                    n2818 = local read "DISP LAB04-2"() -> (w5275:T4)
                    n2819 = local read "DISP LAB04-1"() -> (w5276:T4)
                    n2820 = local read "DISP LAB05-1"() -> (w5274:T4)
                    n2821 = local read "DISP LAB05-2"() -> (w5273:T4)
                    n2822 = Unbundle(w5281) -> ("CYCLE"=w5265:dbl, "MINS"=w5264:dbl, "STATUS"=w5261:string)
                    n2823 = Unbundle(w5282) -> ("CYCLE"=w5270:dbl, "MINS"=w5269:dbl, "STATUS"=w5266:string)
                    n2824 = Unbundle(w5280) -> ("CYCLE"=w5258:dbl, "MINS"=w5257:dbl, "STATUS"=w5256:string)
                    n2825 = Unbundle(w5277) -> ("CYCLE"=w5245:dbl, "MINS"=w5244:dbl, "STATUS"=w5241:string)
                    n2826 = Unbundle(w5278) -> ("CYCLE"=w5250:dbl, "MINS"=w5249:dbl, "STATUS"=w5246:string)
                    n2827 = Unbundle(w5279) -> ("CYCLE"=w5255:dbl, "MINS"=w5254:dbl, "STATUS"=w5251:string)
                    n2828 = Unbundle(w5276) -> ("CYCLE"=w5240:dbl, "MINS"=w5239:dbl, "STATUS"=w5236:string)
                    n2829 = Unbundle(w5275) -> ("CYCLE"=w5235:dbl, "MINS"=w5234:dbl, "STATUS"=w5231:string)
                    n2830 = Unbundle(w5274) -> ("CYCLE"=w5230:dbl, "MINS"=w5229:dbl, "STATUS"=w5226:string)
                    n2831 = Unbundle(w5273) -> ("CYCLE"=w5272:dbl, "MINS"=w5271:dbl, "STATUS"=w5223:string)
                    n2832 = Number To Decimal String(number=w5258) -> (decimal integer string=w5260:string)  [unwired: 1 in]
                    n2833 = Number To Decimal String(number=w5255) -> (decimal integer string=w5253:string)  [unwired: 1 in]
                    n2834 = Number To Decimal String(number=w5250) -> (decimal integer string=w5248:string)  [unwired: 1 in]
                    n2835 = Number To Decimal String(number=w5265) -> (decimal integer string=w5263:string)  [unwired: 1 in]
                    n2836 = Number To Decimal String(number=w5245) -> (decimal integer string=w5243:string)  [unwired: 1 in]
                    n2837 = Number To Decimal String(number=w5270) -> (decimal integer string=w5268:string)  [unwired: 1 in]
                    n2838 = Number To Decimal String(number=w5272) -> (decimal integer string=w5225:string)  [unwired: 1 in]
                    n2839 = Number To Decimal String(number=w5240) -> (decimal integer string=w5238:string)  [unwired: 1 in]
                    n2840 = Number To Decimal String(number=w5235) -> (decimal integer string=w5233:string)  [unwired: 1 in]
                    n2841 = Number To Decimal String(number=w5230) -> (decimal integer string=w5228:string)  [unwired: 1 in]
                    n2842 = Number To Fractional String(number=w5257, precision (6)=w5202) -> (F-format string=w5259:string)  [unwired: 2 in]
                    n2843 = Number To Fractional String(number=w5244, precision (6)=w5202) -> (F-format string=w5242:string)  [unwired: 2 in]
                    n2844 = Number To Fractional String(number=w5254, precision (6)=w5202) -> (F-format string=w5252:string)  [unwired: 2 in]
                    n2845 = Number To Fractional String(number=w5249, precision (6)=w5202) -> (F-format string=w5247:string)  [unwired: 2 in]
                    n2846 = Number To Fractional String(number=w5234, precision (6)=w5202) -> (F-format string=w5232:string)  [unwired: 2 in]
                    n2847 = Number To Fractional String(number=w5239, precision (6)=w5202) -> (F-format string=w5237:string)  [unwired: 2 in]
                    n2848 = Number To Fractional String(number=w5264, precision (6)=w5202) -> (F-format string=w5262:string)  [unwired: 2 in]
                    n2849 = Number To Fractional String(number=w5229, precision (6)=w5202) -> (F-format string=w5227:string)  [unwired: 2 in]
                    n2850 = Number To Fractional String(number=w5269, precision (6)=w5202) -> (F-format string=w5267:string)  [unwired: 2 in]
                    n2851 = Number To Fractional String(number=w5271, precision (6)=w5202) -> (F-format string=w5224:string)  [unwired: 2 in]
                    n2852 = Concatenate Strings(w5201, w5243, w5201, w5242, w5201, w5241) -> (w5217:string)
                    n2853 = Concatenate Strings(w5201, w5238, w5201, w5237, w5201, w5236) -> (w5216:string)
                    n2854 = Concatenate Strings(w5201, w5233, w5201, w5232, w5201, w5231) -> (w5215:string)
                    n2855 = Concatenate Strings(w5201, w5228, w5201, w5227, w5201, w5226) -> (w5214:string)
                    n2856 = Concatenate Strings(w5201, w5225, w5201, w5224, w5201, w5223) -> (w5213:string)
                    n2857 = Concatenate Strings(w5201, w5268, w5201, w5267, w5201, w5266) -> (w5222:string)
                    n2858 = Concatenate Strings(w5201, w5248, w5201, w5247, w5201, w5246) -> (w5218:string)
                    n2859 = Concatenate Strings(w5201, w5263, w5201, w5262, w5201, w5261) -> (w5221:string)
                    n2860 = Concatenate Strings(w5201, w5260, w5201, w5259, w5201, w5256) -> (w5220:string)
                    n2861 = Concatenate Strings(w5201, w5253, w5201, w5252, w5201, w5251) -> (w5219:string)
                    n2862 = Concatenate Strings("]", "\r") -> (w5198:string)
                    n2863 = Concatenate Strings(w5193, w5218, w5198) -> (w5208:string)
                    n2864 = Concatenate Strings(w5195, w5220, w5198) -> (w5210:string)
                    n2865 = Concatenate Strings(w5194, w5219, w5198) -> (w5209:string)
                    n2866 = Concatenate Strings(w5190, w5215, w5198) -> (w5205:string)
                    n2867 = Concatenate Strings(w5191, w5214, w5198) -> (w5206:string)
                    n2868 = Concatenate Strings(w5189, w5216, w5198) -> (w5204:string)
                    n2869 = Concatenate Strings(w5188, w5217, w5198) -> (w5203:string)
                    n2870 = Concatenate Strings(w5192, w5213, w5198) -> (w5207:string)
                    n2871 = Concatenate Strings(w5196, w5221, w5198) -> (w5211:string)
                    n2872 = Concatenate Strings(w5197, w5222, w5198) -> (w5212:string)
                    n2873 = Concatenate Strings(w5212, w5211, w5210, w5209, w5208, w5203, w5204, w5205, w5206, w5207) -> (w5181:string)
                    n2874 = Concatenate Strings("[PANEL/", "DESC/", "CYCLES/", "MINS/", "STATUS]", "\r", w5181) -> (w5180:string)
                    "MAIL REPORT" <- w5180
                    n2875 = global write "Global display 3.vi" "log all"(w5180) -> ()
                  }
                  frame #2 {
                    w5311 = "END"
                    n2876 = local read "mail control"() -> (w5312:string)
                    n2877 = case shown="False" w5307 {
                      tunnel: w5312 -> [w5336 _]
                      tunnel: w5311 -> [w5335 _]
                      tunnel: [w5334 FALSE] -> w5297
                      frame False {
                        n2878 = Equal?(x=w5336, y=w5335) -> (x = y?=w5334:bool)
                      }
                      frame True {
                      }
                    }
                    n2879 = case shown="False" w5313 {
                      tunnel: w5312 -> [w5352 _]
                      tunnel: w5311 -> [w5351 _]
                      tunnel: [w5350 FALSE] -> w5301
                      frame False {
                        n2880 = Equal?(x=w5352, y=w5351) -> (x = y?=w5350:bool)
                      }
                      frame True {
                      }
                    }
                    n2881 = case shown="False" w5310 {
                      tunnel: w5312 -> [w5348 _]
                      tunnel: w5311 -> [w5347 _]
                      tunnel: [w5346 FALSE] -> w5300
                      frame False {
                        n2882 = Equal?(x=w5348, y=w5347) -> (x = y?=w5346:bool)
                      }
                      frame True {
                      }
                    }
                    n2883 = case shown="False" w5308 {
                      tunnel: w5312 -> [w5340 _]
                      tunnel: w5311 -> [w5339 _]
                      tunnel: [w5338 FALSE] -> w5298
                      frame False {
                        n2884 = Equal?(x=w5340, y=w5339) -> (x = y?=w5338:bool)
                      }
                      frame True {
                      }
                    }
                    n2885 = case shown="False" w5309 {
                      tunnel: w5312 -> [w5344 _]
                      tunnel: w5311 -> [w5343 _]
                      tunnel: [w5342 FALSE] -> w5299
                      frame False {
                        n2886 = Equal?(x=w5344, y=w5343) -> (x = y?=w5342:bool)
                      }
                      frame True {
                      }
                    }
                    n2887 = Or(x=w5299, y=w5298) -> (x .or. y?=w5290:bool)
                    n2888 = Or(x=w5301, y=w5300) -> (x .or. y?=w5291:bool)
                    n2889 = Or(x=w5291, y=w5290) -> (x .or. y?=w5286:bool)
                    n2890 = case shown="False" w5303 {
                      tunnel: w5312 -> [w5320 _]
                      tunnel: w5311 -> [w5319 _]
                      tunnel: [w5318 FALSE] -> w5292
                      frame False {
                        n2891 = Equal?(x=w5320, y=w5319) -> (x = y?=w5318:bool)
                      }
                      frame True {
                      }
                    }
                    n2892 = case shown="False" w5302 {
                      tunnel: w5312 -> [w5316 _]
                      tunnel: w5311 -> [w5315 _]
                      tunnel: [w5314 FALSE] -> w5296
                      frame False {
                        n2893 = Equal?(x=w5316, y=w5315) -> (x = y?=w5314:bool)
                      }
                      frame True {
                      }
                    }
                    n2894 = case shown="False" w5304 {
                      tunnel: w5312 -> [w5324 _]
                      tunnel: w5311 -> [w5323 _]
                      tunnel: [w5322 FALSE] -> w5293
                      frame False {
                        n2895 = Equal?(x=w5324, y=w5323) -> (x = y?=w5322:bool)
                      }
                      frame True {
                      }
                    }
                    n2896 = case shown="False" w5306 {
                      tunnel: w5312 -> [w5332 _]
                      tunnel: w5311 -> [w5331 _]
                      tunnel: [w5330 FALSE] -> w5295
                      frame False {
                        n2897 = Equal?(x=w5332, y=w5331) -> (x = y?=w5330:bool)
                      }
                      frame True {
                      }
                    }
                    n2898 = case shown="False" w5305 {
                      tunnel: w5312 -> [w5328 _]
